vi "orderbook.test.2.vi"(8 "error in":errorcluster) -> (0 "error out":errorcluster, 3 "Passed":bool)   [LabVIEW 2020]
uses:
  arty/orderbook/orderbook.command.ctl
  arty/orderbook/orderbook.command.type.ctl
  arty/application/orderbook.entry.ctl
  arty/application/orderbook.result.type.ctl
panel:
  out "OrderBook.Entries":T1[](array[typedef])
  out "output cluster":T3
  in  "OrderBook.Command[]\nto Send":T4[](array[typedef])=[{"OrderBook Command.Type"=enum."AddOrder", "Side (U8)"=66, "Order Id (U64)"=0, "Quantity (U32)"=125, "Symbol (U64)"=29033, "Price (U64)"=9811, "Executed Quantity (U32)"=0, "Cancelled Quantity (U32)"=0}, {"OrderBook Command.Type"=enum."Query", "Side (U8)"=0, "Order Id (U64)"=0, "Quantity (U32)"=0, "Symbol (U64)"=29033, "Price (U64)"=0, "Executed Quantity (U32)"=0, "Cancelled Quantity (U32)"=0}] {"Side (U8)" format="%.0x"; "Order Id (U64)" format="%.0x"; "Symbol (U64)" format="%.0x"}
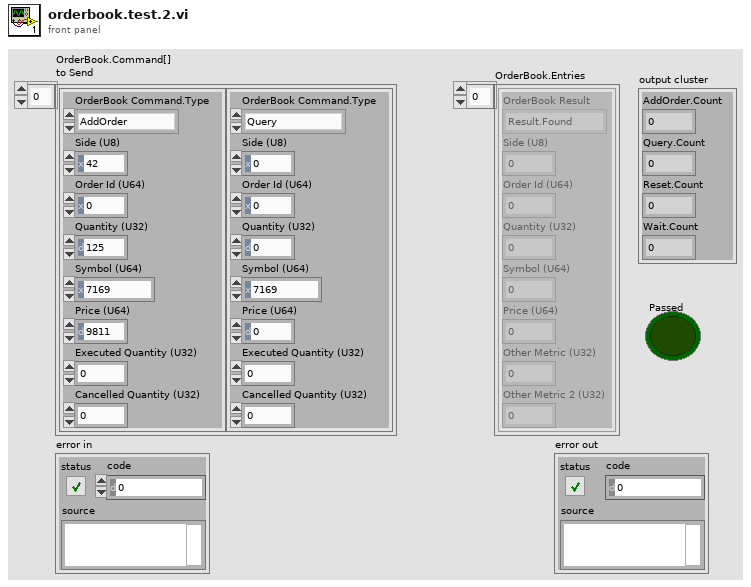
[diagram p1: front panel]
types:
  T1 = typedef "orderbook.entry.ctl" = cluster{"OrderBook Result":T2, "Side (U8)":u8, "Order Id (U64)":u64, "Quantity (U32)":u32, "Symbol (U64)":u64, "Price (U64)":u64, "Other Metric (U32)":u32, "Other Metric 2 (U32)":u32}
  T2 = typedef "orderbook.result.type.ctl" = enum16{"Result.Found", "Result.Not.Found"}
  T3 = cluster{"AddOrder.Count":u32, "Query.Count":u32, "Reset.Count":u32, "Wait.Count":u32}
  T4 = typedef "orderbook.command.ctl" = cluster{"OrderBook Command.Type":T5, "Side (U8)":u8, "Order Id (U64)":u64, "Quantity (U32)":u32, "Symbol (U64)":u64, "Price (U64)":u64, "Executed Quantity (U32)":u32, "Cancelled Quantity (U32)":u32}
  T5 = typedef "orderbook.command.type.ctl" = enum16{"AddOrder", "OrderExecuted", "ReduceSize", "ModifyOrder", "DeleteOrder", "Query"}
  T6 = cluster{"Write.Request":bool, "Read.Request":bool, "Read.Address":u32, "Read.OrderBook.Entry":cluster{"OrderBook Result":enum16{"Result.Found", "Result.Not.Found"}, "Side (U8)":u8, "Order Id (U64)":u64, "Quantity (U32)":u32, "Symbol (U64)":u64, "Price (U64)":u64, "Other Metric (U32)":u32, "Other Metric 2 (U32)":u32}, "Number.of.Entries":u32, "OrderBook.State":enum16{"Reset", "WaitForNewCommand", "AddOrder", "Query"}, "Ready.For.OrderBook.Command":bool, "Memory.State":enum16{"New", "Request.Data", "Append", "Data.Ready"}, "Move":bool, "Read.Valid":bool, "Write.Address":u32, "Write.OrderBook.Entry":cluster{"OrderBook Result":enum16{"Result.Found", "Result.Not.Found"}, "Side (U8)":u8, "Order Id (U64)":u64, "Quantity (U32)":u32, "Symbol (U64)":u64, "Price (U64)":u64, "Other Metric (U32)":u32, "Other Metric 2 (U32)":u32}, "OrderBook.Result.Valid":bool, "AddOrder.Count":u32, "Query.Count":u32, "Reset.Count":u32, "Wait.Count":u32, "Append":bool}
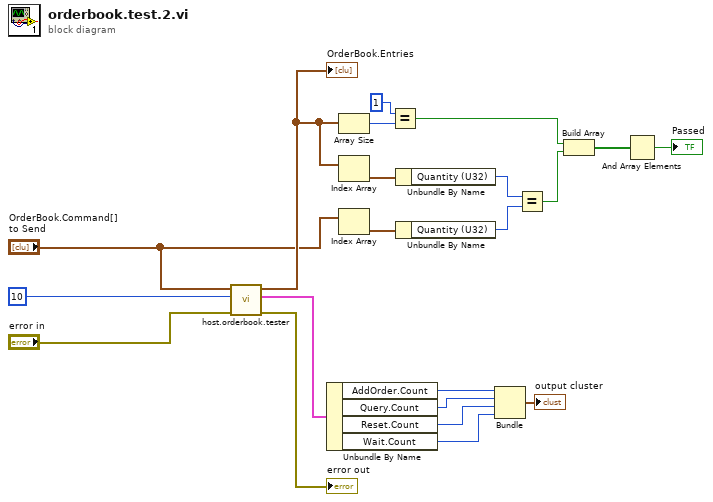
[diagram p0: block diagram]
diagram:
  n1 = call "host.orderbook.tester.vi"("error in"="error in", "Seconds to Wait"=10 ("Seconds\nto\nWait"), "OrderBook.Command[]\nto Send"="OrderBook.Command[]\nto Send") -> ("error out"=→"error out":errorcluster, "OrderBook.Variables"=w13:T6, "OrderBook.Entries"=w10:T1[])  [unwired: 6 in]
  "OrderBook.Entries" <- w10
  n2 = Unbundle By Name(w13) -> ("AddOrder.Count"=w18:u32, "Query.Count"=w15:u32, "Reset.Count"=w16:u32, "Wait.Count"=w17:u32)
  n3 = Array Size(array=w10) -> (size(s)=w12:i32)
  n4 = Index Array(array=w10) -> (element=w9:T1)  [unwired: 1 in]
  n5 = Index Array(array="OrderBook.Command[]\nto Send") -> (element=w7:T4)  [unwired: 1 in]
  n6 = Equal?(x=1, y=w12) -> (x = y?=w3:bool)
  n7 = Unbundle By Name(w9) -> ("Quantity (U32)"=w6:u32)
  n8 = Unbundle By Name(w7) -> ("Quantity (U32)"=w5:u32)
  n9 = Bundle("AddOrder.Count"=w18, "Query.Count"=w15, "Reset.Count"=w16, "Wait.Count"=w17) -> (→"output cluster":T3)  [unwired: 1 in]
  n10 = Equal?(x=w6, y=w5) -> (x = y?=w4:bool)
  n11 = Build Array(w3, w4) -> (w2:bool[])
  n12 = And Array Elements(Boolean array=w2) -> (logical AND=→"Passed":bool)
